vi "EOL CAN_Send_Two_Part_Message.vi"(9 "Tx 2":u8[](array[numeric])=[48, 8, 40, 255, 255, 255, 255, 255] format="%02x", 10 "Tx 1":u8[](array[numeric])=[2, 26, 156, 255, 255, 255, 255, 255] format="%02x", 11 "NetworkObjHandle":T1) -> (0 "Array 23":u8[](array[numeric]) format="%02x", 1 "Array 22":u8[](array[numeric]) format="%02x", 2 "Array 21":u8[](array[numeric]) format="%02x", 3 "Response Good?":bool, 5 "TxRx Data":string[][](array[string]))   [LabVIEW 2018]
uses:
  <vilib>/nican/nican.llb/xobjhandle.ctl
panel:
  in  "Arbitration Id 2":u32=1592 format="%04x"
  in  "Arbitration Id 1":u32=1592 format="%04x"
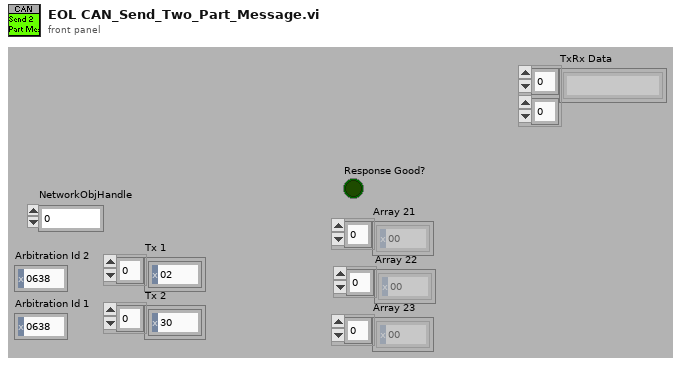
[diagram p1: front panel]
types:
  T1 = typedef "xobjhandle.ctl" = u32
  T2 = cluster{"NetworkObjHandle":T1, "Retry Counter":i32, "Array 21":u8[], "Array 22":u8[], "Array 23":u8[], "Response Good?":bool, "TxRx Data":string[][]}
  T3 = typedef "CanFrameTimed.ctl" = cluster{"Timestamp":dbl, "ArbitrationId":u32, "IsRemote":u8, "DataLength":u8, "Data":u8[]}
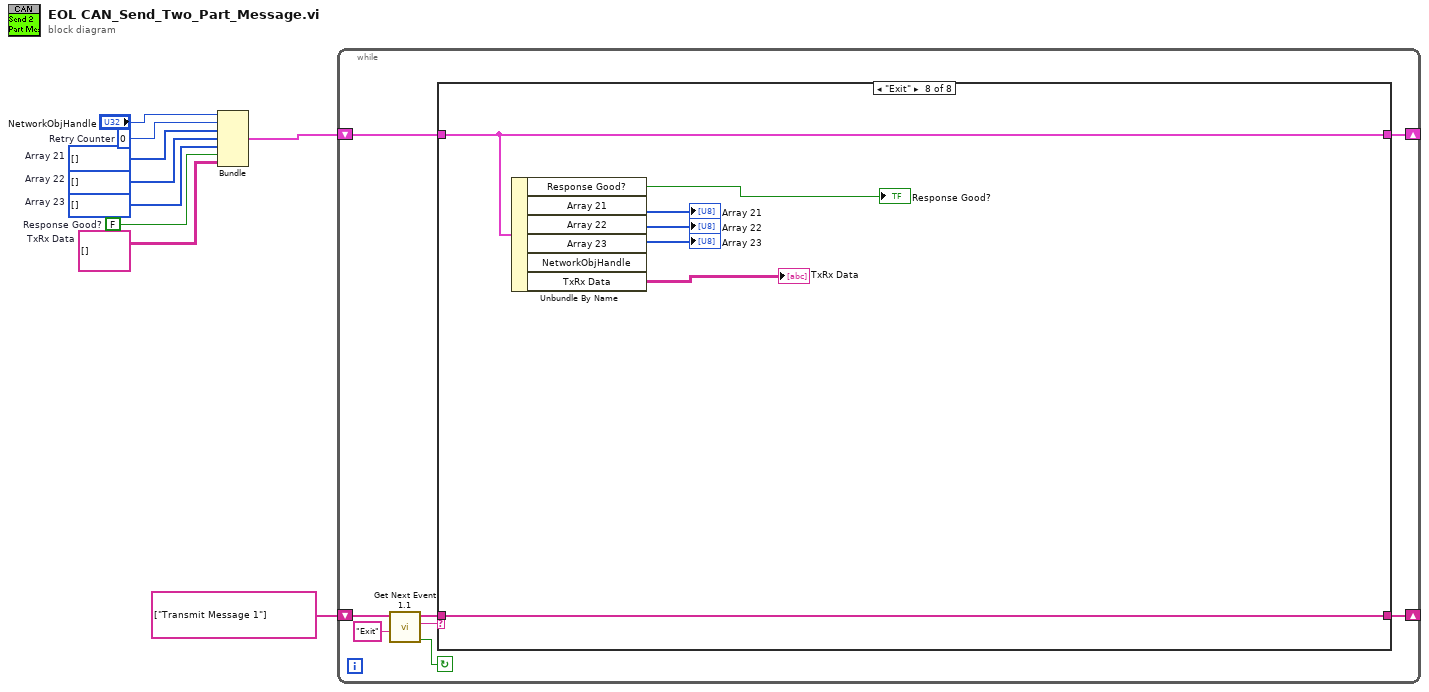
[diagram p0: block diagram]
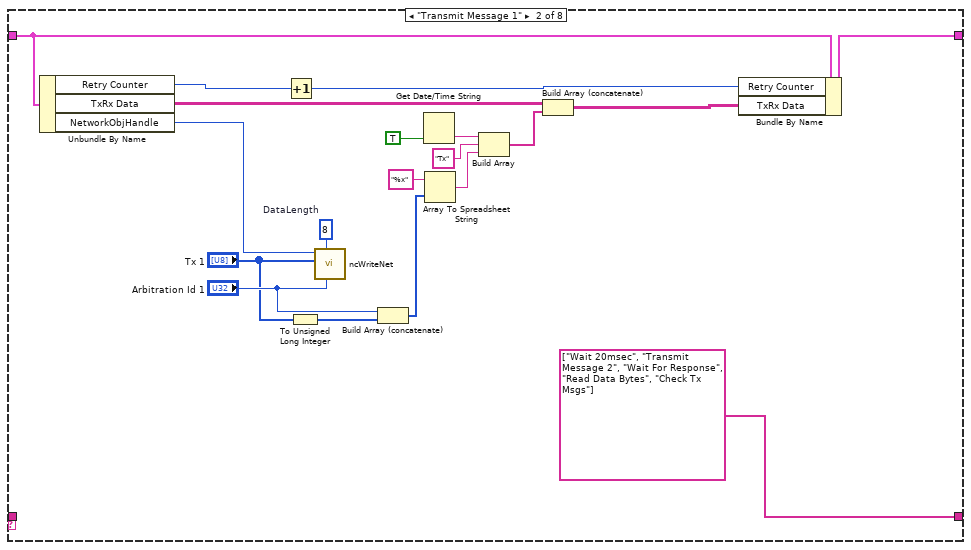
[diagram p3: hidden frame]
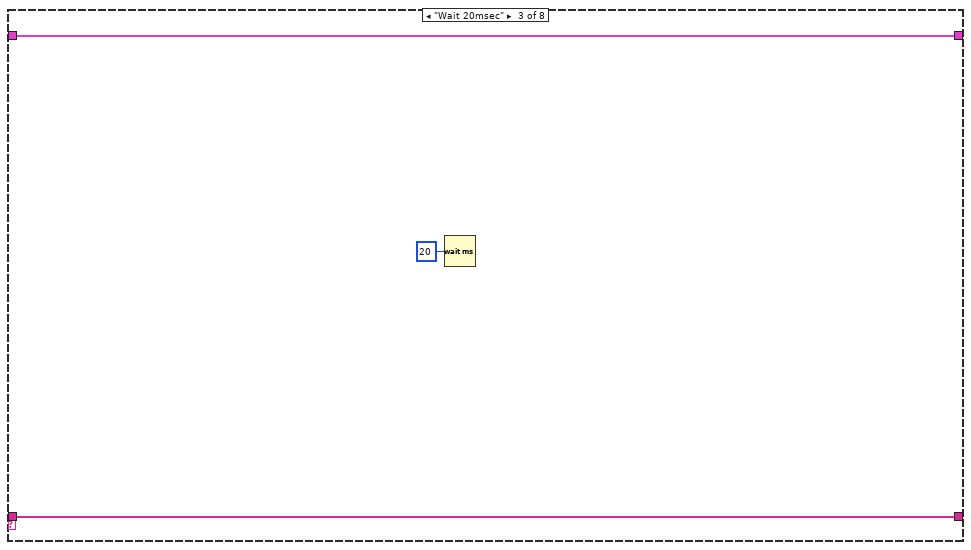
[diagram p4: hidden frame]
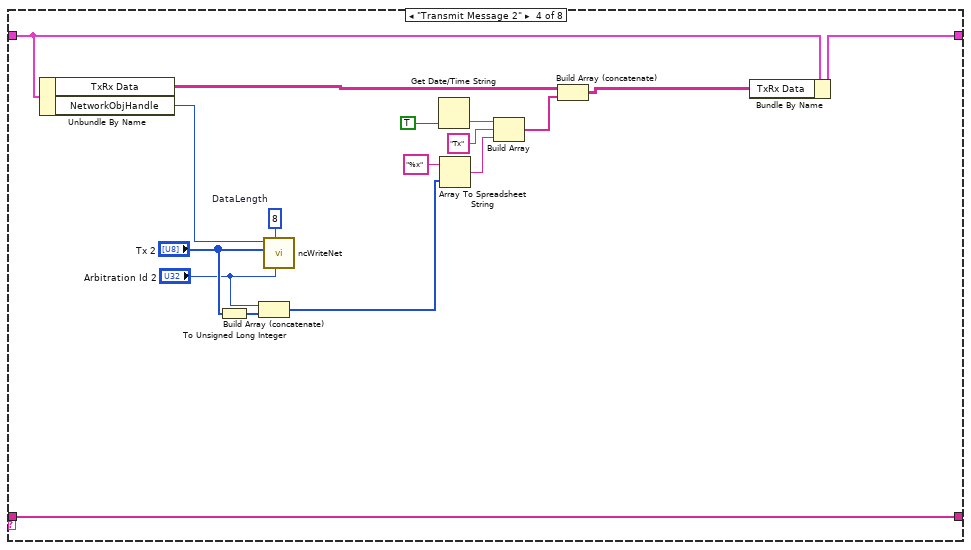
[diagram p5: hidden frame]
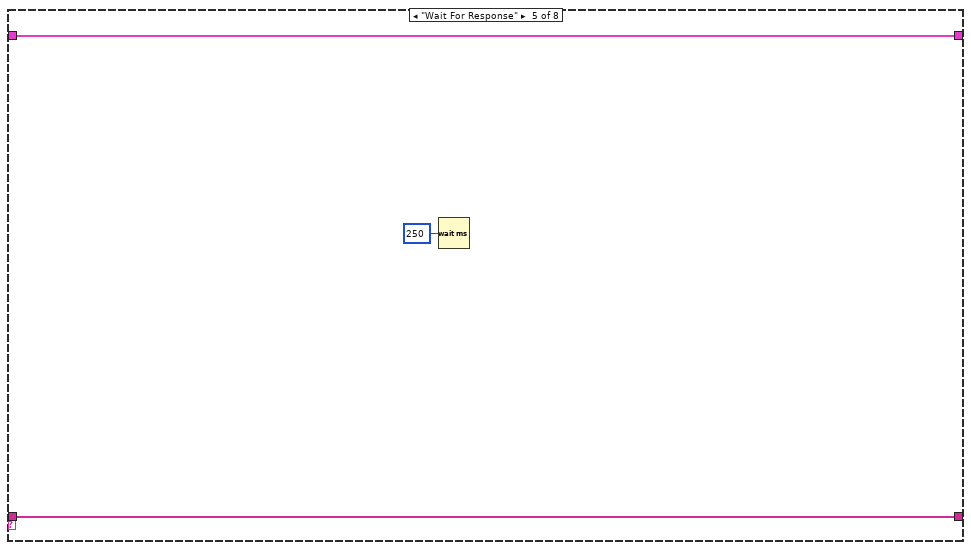
[diagram p6: hidden frame]
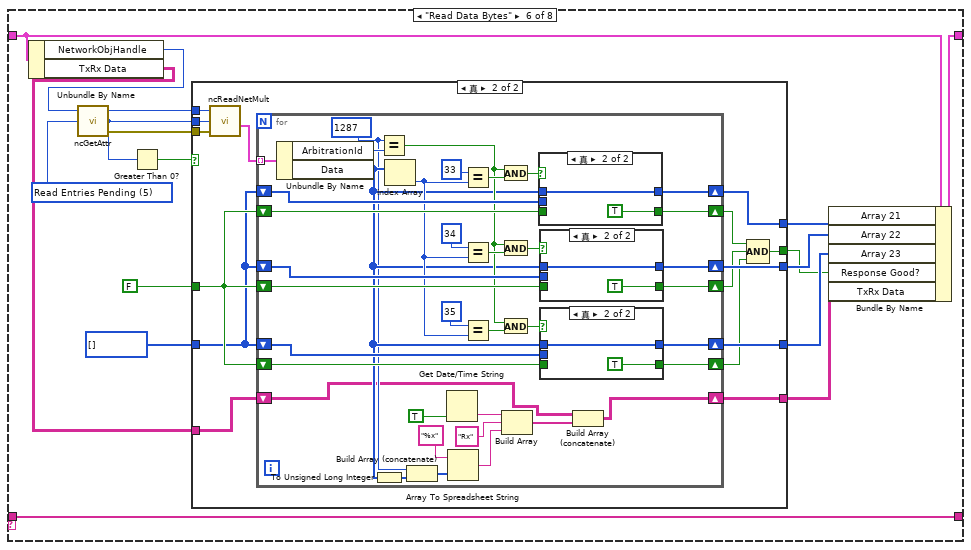
[diagram p7: hidden frame]
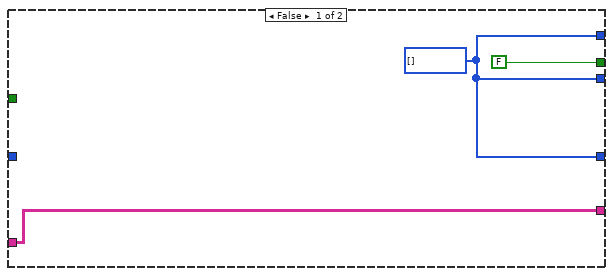
[diagram p8: hidden frame]
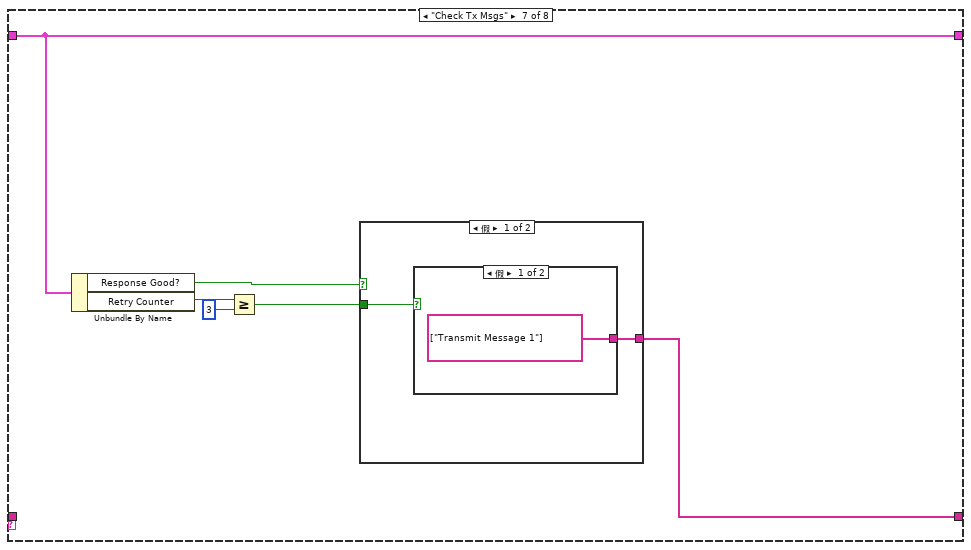
[diagram p12: hidden frame]
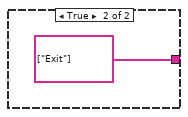
[diagram p13: hidden frame]
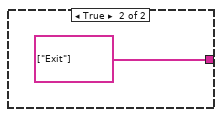
[diagram p14: hidden frame]
diagram:
  w1 = string[][] []  # TxRx Data
  w3 = FALSE  # Response Good?
  w4 = u8[] []  # Array 23
  w5 = u8[] []  # Array 22
  w6 = u8[] []  # Array 21
  w8 = 0  # Retry Counter
  n1 = Bundle("NetworkObjHandle"="NetworkObjHandle", "Retry Counter"=w8, "Array 21"=w6, "Array 22"=w5, "Array 23"=w4, "Response Good?"=w3, "TxRx Data"=w1) -> (w7:T2)  [unwired: 1 in]
  n2 = while {
    shift-right: [w14] -> _
    shift-left: string[] ["Transmit Message 1"] ("event queue out") -> [w13]
    shift-right: [w11] -> _
    shift-left: w7 -> [w12]
    stop <- w17 continue-if-true
    n3 = call "Get Next Event 1.1.vi"("Exit Event"="Exit", "event queue in"=w13) -> ("Condition (Exit:F)"=w17:bool, "next event"=w16:string, "event queue out"=w15:string[])  [unwired: 6 in, 1 out]
    n4 = case shown="\"Exit\"" w16 {
      tunnel: w15 -> [w19 _ w41 w52 w59 w64 _ w163]
      tunnel: [w19 string[] ["Wait 20msec", "Transmit Message 2", "Wait For Response", "Read Data Bytes", "Check Tx Msgs"] ("event queue out") w41 w52 w59 w64 w148 w163] -> w14
      tunnel: w12 -> [w18 w36 w40 w58 w60 w73 w146 w162]
      tunnel: [w18 w34 w40 w57 w60 w72 w146 w162] -> w11
      frame "Error", Default {
      }
      frame "Transmit Message 1" {
        w32 = u32 8  # DataLength
        n5 = Unbundle By Name(w36) -> ("Retry Counter"=w37:i32, "TxRx Data"=w21:string[][], "NetworkObjHandle"=w33:T1)
        n6 = Increment(x=w37) -> (x+1=w35:i32)
        n7 = To Unsigned Long Integer(number="Tx 1") -> (unsigned 32bit integer=w29:u32[])
        n8 = call <vilib>:"ncWriteNet.vi"("ArbitrationId"="Arbitration Id 1", "DataLength"=w32, "Data"="Tx 1", "ObjHandle in"=w33) -> ()  [unwired: 2 in, 2 out]
        n9 = Build Array (concatenate)("Arbitration Id 1", w29) -> (w22:u32[])
        n10 = Get Date/Time String(want seconds? (F)=TRUE) -> (time string=w25:string)  [unwired: 2 in, 1 out]
        n11 = Array To Spreadsheet String(array=w22, 3:"%x" ("format string")) -> (spreadsheet string=w27:string)  [unwired: 1 in]
        n12 = Build Array(w25, "Tx" ("format string"), w27) -> (w28:string[])
        n13 = Build Array (concatenate)(w21, w28) -> (w20:string[][])
        n14 = Bundle By Name(cluster=w36, "Retry Counter"=w35, "TxRx Data"=w20) -> (w34:T2)
      }
      frame "Wait 20msec" {
        n15 = Wait (ms)(milliseconds to wait=u32 20) -> ()  [unwired: 1 out]
      }
      frame "Transmit Message 2" {
        w56 = u32 8  # DataLength
        n16 = Unbundle By Name(w58) -> ("TxRx Data"=w44:string[][], "NetworkObjHandle"=w55:T1)
        n17 = To Unsigned Long Integer(number="Tx 2") -> (unsigned 32bit integer=w51:u32[])
        n18 = Build Array (concatenate)("Arbitration Id 2", w51) -> (w42:u32[])
        n19 = call <vilib>:"ncWriteNet.vi"("ArbitrationId"="Arbitration Id 2", "DataLength"=w56, "Data"="Tx 2", "ObjHandle in"=w55) -> ()  [unwired: 2 in, 2 out]
        n20 = Get Date/Time String(want seconds? (F)=TRUE) -> (time string=w47:string)  [unwired: 2 in, 1 out]
        n21 = Array To Spreadsheet String(array=w42, 3:"%x" ("format string")) -> (spreadsheet string=w49:string)  [unwired: 1 in]
        n22 = Build Array(w47, "Tx" ("format string"), w49) -> (w50:string[])
        n23 = Build Array (concatenate)(w44, w50) -> (w43:string[][])
        n24 = Bundle By Name(cluster=w58, "TxRx Data"=w43) -> (w57:T2)
      }
      frame "Wait For Response" {
        n25 = Wait (ms)(milliseconds to wait=u32 250) -> ()  [unwired: 1 out]
      }
      frame "Read Data Bytes" {
        w76 = u32 5 items=["(reserved)", "Protocol Version", "Software Version", "Object State", "(reserved)", "Read Entries Pending", "Write Entries Pending", "ReadMult Size for Notification", "Listen Only?", "Self Reception?", "Transmit Error Counter", "Receive Error Counter", "Single Shot Transmit?", "Series 2 Filter Mode", "Series 2 Mask", "Series 2 Comparator", "Serial Number", "Form Factor", "Series", "Transceiver Type", "Interface Number", "Series 2 Error/Arb Capture", "Transceiver Mode", "Transceiver External Outputs", "Transceiver External Inputs", "Start Trigger Behavior", "Log Comm Warnings", "User RTSI Frame", "Transmit Mode", "Log Start Trigger?", "Timestamp Format", "Master Timebase Rate", "Virtual Bus Timing"] ("AttrId")
        n26 = Unbundle By Name(w73) -> ("NetworkObjHandle"=w65:T1, "TxRx Data"=w63:string[][])
        n27 = call <vilib>:"ncGetAttr.vi"("AttrId"=w76, "ObjHandle in"=w65) -> ("Error out"=w78:errorcluster, "AttrValue"=w74:u32, "ObjHandle out"=w77:T1)  [unwired: 1 in]
        n28 = Greater Than 0?(x=w74) -> (x > 0?=w75:bool)
        n29 = case shown="真" w75 {
          tunnel: w74 -> [_ w96]
          tunnel: w78 -> [_ w95]
          tunnel: w77 -> [_ w94]
          tunnel: [FALSE w90] -> w66
          tunnel: [w80 w92] -> w71
          tunnel: u8[] [] ("Data Array") -> [_ w85]
          tunnel: FALSE -> [_ w86]
          tunnel: [w80 w89] -> w68
          tunnel: [w80 w87] -> w67
          tunnel: w63 -> [w79 w83]
          tunnel: [w79 w82] -> w62
          frame False {
            w80 = u8[] [] ("Data Array")
          }
          frame True {
            n30 = call <vilib>:"ncReadNetMult.vi"("ObjHandle in"=w94, "Requested Number of Frames"=w96, "Error in"=w95) -> ("Data"=w93:T3[])  [unwired: 3 out]
            n31 = for {
              tunnel: w93 -> [w133] mode=indexing
              shift-right: [w131] -> w92
              shift-left: w85 -> [w130]
              shift-right: [w129] -> w91
              shift-left: w86 -> [w128]
              shift-right: [w125] -> w88
              shift-left: w86 -> [w118]
              shift-right: [w124] -> w89
              shift-left: w85 -> [w123]
              shift-right: [w111] -> w84
              shift-left: w86 -> [w117]
              shift-right: [w112] -> w87
              shift-left: w85 -> [w113]
              shift-right: [w98] -> w82
              shift-left: w83 -> [w97]
              w100 = u32 1287 ("x")
              n32 = Unbundle By Name(w133) -> ("ArbitrationId"=w132:u32, "Data"=w102:u8[])
              n33 = To Unsigned Long Integer(number=w102) -> (unsigned 32bit integer=w99:u32[])
              n34 = Equal?(x=w100, y=w132) -> (x = y?=w109:bool)
              n35 = Index Array(array=w102) -> (element=w110:u8)  [unwired: 1 in]
              n36 = Build Array (concatenate)(w100, w99) -> (w101:u32[])
              n37 = Get Date/Time String(want seconds? (F)=TRUE) -> (time string=w105:string)  [unwired: 2 in, 1 out]
              n38 = Array To Spreadsheet String(array=w101, 3:"%x" ("format string")) -> (spreadsheet string=w107:string)  [unwired: 1 in]
              n39 = Equal?(x=u8 33 ("y"), y=w110) -> (x = y?=w126:bool)
              n40 = Equal?(x=u8 34 ("y"), y=w110) -> (x = y?=w122:bool)
              n41 = Equal?(x=u8 35 ("y"), y=w110) -> (x = y?=w114:bool)
              n42 = And(x=w109, y=w126) -> (x .and. y?=w127:bool)
              n43 = And(x=w109, y=w122) -> (x .and. y?=w121:bool)
              n44 = And(x=w109, y=w114) -> (x .and. y?=w115:bool)
              n45 = Build Array(w105, "Rx" ("format string"), w107) -> (w108:string[])
              n46 = case shown="真" w127 {
                tunnel: w102 -> [_ w144]
                tunnel: [w143 w144] -> w131
                tunnel: w130 -> [w143 _]
                tunnel: [w142 TRUE] -> w129
                tunnel: w128 -> [w142 _]
                frame False {
                }
                frame True {
                }
              }
              n47 = case shown="真" w121 {
                tunnel: w102 -> [_ w140]
                tunnel: [w139 w140] -> w124
                tunnel: w123 -> [w139 _]
                tunnel: [w138 TRUE] -> w125
                tunnel: w118 -> [w138 _]
                frame False {
                }
                frame True {
                }
              }
              n48 = case shown="真" w115 {
                tunnel: w102 -> [_ w136]
                tunnel: [w135 w136] -> w112
                tunnel: w113 -> [w135 _]
                tunnel: [w134 TRUE] -> w111
                tunnel: w117 -> [w134 _]
                frame False {
                }
                frame True {
                }
              }
              n49 = Build Array (concatenate)(w97, w108) -> (w98:string[][])
            }
            n50 = Compound Arithmetic op=AND(w91, w88, w84) -> (w90:bool)
          }
        }
        n51 = Bundle By Name(cluster=w73, "Array 21"=w71, "Array 22"=w68, "Array 23"=w67, "Response Good?"=w66, "TxRx Data"=w62) -> (w72:T2)
      }
      frame "Check Tx Msgs" {
        n52 = Unbundle By Name(w146) -> ("Response Good?"=w149:bool, "Retry Counter"=w150:i32)
        n53 = Greater Or Equal?(x=w150, y=3) -> (x >= y?=w147:bool)
        n54 = case shown="假" w149 {
          tunnel: [w152 string[] ["Exit"] ("event queue out")] -> w148
          tunnel: w147 -> [w153 _]
          frame False {
            n55 = case shown="假" w153 {
              tunnel: [string[] ["Transmit Message 1"] ("f") string[] ["Exit"] ("event queue out")] -> w152
              frame False {
              }
              frame True {
              }
            }
          }
          frame True {
          }
        }
      }
      frame "Exit" {
        n56 = Unbundle By Name(w162) -> ("Response Good?"=→"Response Good?":bool, "Array 21"=→"Array 21":u8[], "Array 22"=→"Array 22":u8[], "Array 23"=→"Array 23":u8[], "TxRx Data"=→"TxRx Data":string[][])  [unwired: 1 out]
      }
    }
  }
